vi "Create Subscription.vi"(7 "Inbound Message":refnum<user-event>, 8 "error in (no error)":errorcluster, 9 "SessionMailbox":refnum<queue>, 10 "QoS":T1, 11 "Topic Filter":string) -> (0 "error out":errorcluster, 3 "Subscription out":refnum<class "Subscription.lvclass">)   [LabVIEW 2013, in "MQTT Base.lvlib" / "Subscription.lvclass"]
uses:
  Subscription.lvclass
  <vilib>/LabVIEW Open Source Project/MQTT Control Packets/Control Packets/ControlPacket/QualityOfService -- enum.ctl
  Base Class/Response -- cluster.ctl
  <vilib>/LabVIEW Open Source Project/MQTT Control Packets/Control Packets/ControlPacket/ControlPacket.lvclass
  <vilib>/LabVIEW Open Source Project/MQTT Control Packets/Control Packets/PUBLISH/PUBLISH.lvclass
  Queued Message -- cluster.ctl
  Subscription.lvclass/Subscription.ctl
  TopicFilter/TopicFilter.lvclass
  Base Class/MQTT_Base.lvclass
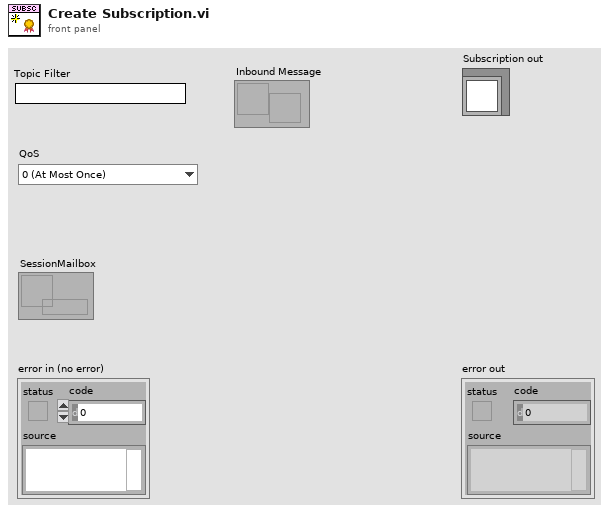
[diagram p1: front panel]
types:
  T1 = typedef "MQTT_Control_Packets.lvlib/ControlPacket.lvclass/QualityOfService -- enum.ctl" = enum16{"0 (At Most Once)", "1 (At Least Once)", "2 (Exactly Once)"}
  T2 = typedef "MQTT Base.lvlib/Subscription.lvclass/Queued Message -- cluster.ctl" = cluster{"Message":refnum<class "PUBLISH.lvclass">, "PUBREC received":bool}
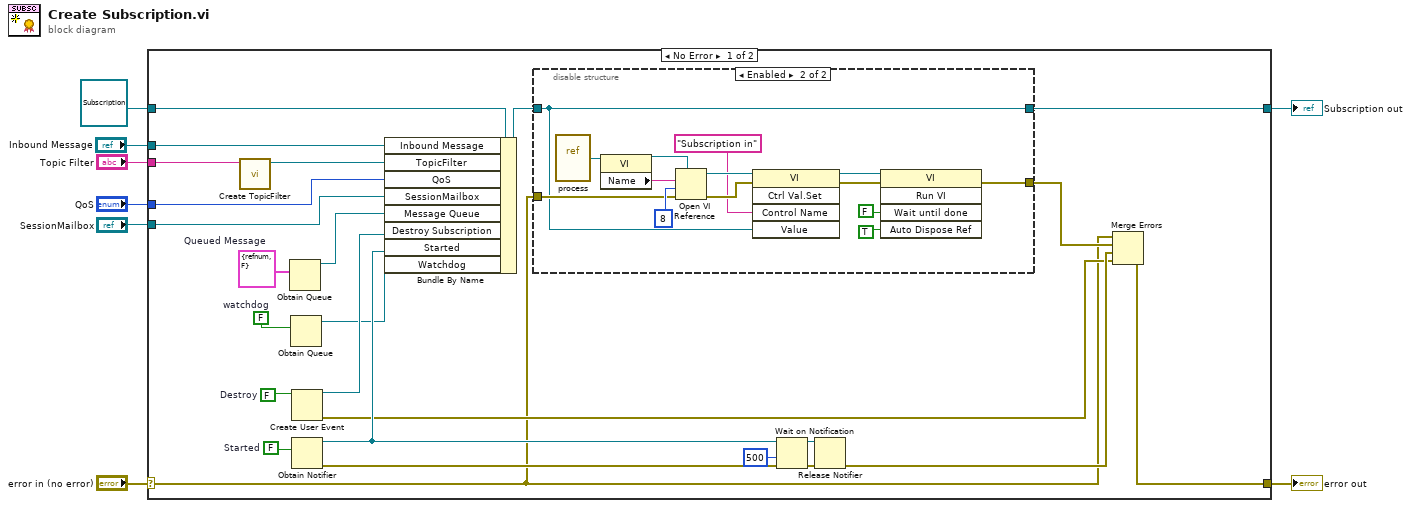
[diagram p0: block diagram]
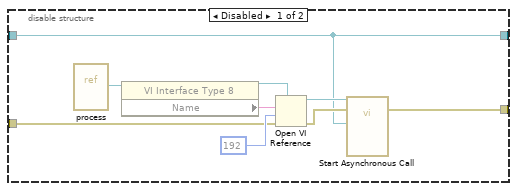
[diagram p2: hidden frame]
diagram:
  n1 = case shown="No Error" "error in (no error)" {
    selector: "error in (no error)" -> [w11 w58]
    tunnel: [w20 w58] -> w7
    tunnel: [w12 w57] -> w5
    tunnel: refnum<class "Subscription.lvclass"> refnum ("Subscription in") -> [w31 w57]
    tunnel: "Topic Filter" -> [w19 _]
    tunnel: "QoS" -> [w33 _]
    tunnel: "SessionMailbox" -> [w32 _]
    tunnel: "Inbound Message" -> [w29 _]
    frame No Error {
      w10 = FALSE  # watchdog
      w17 = FALSE  # Destroy
      w28 = FALSE  # Started
      w30 = T2 {"Message"=refnum, "PUBREC received"=FALSE}  # Queued Message
      n2 = call "Create TopicFilter.vi"("Topic Filter"=w19) -> ("TopicFilter out"=w18:refnum<class "TopicFilter.lvclass">)  [unwired: 9 in, 1 out]
      n3 = Obtain Queue(element data type=w30) -> (queue out=w27:refnum<queue>)  [unwired: 4 in, 2 out]
      n4 = Obtain Queue(element data type=w10) -> (queue out=w9:refnum<queue>)  [unwired: 4 in, 2 out]
      n5 = Create User Event(user event datatype=w17) -> (user event=w16:refnum<user-event>, error out=w15:errorcluster)  [unwired: 1 in]
      n6 = Obtain Notifier(notification data type=w28) -> (notifier out=w26:refnum<notifier>, error out=w23:errorcluster)  [unwired: 3 in, 1 out]
      n7 = Bundle By Name(cluster=w31, "Inbound Message"=w29, "TopicFilter"=w18, "QoS"=w33, "SessionMailbox"=w32, "Message Queue"=w27, "Destroy Subscription"=w16, "Started"=w26, "Watchdog"=w9) -> (w13:refnum<class "Subscription.lvclass">)
      n8 = disable-structure shown="Enabled" {
        disable-tunnel: w11 -> [w37 w53]
        disable-tunnel: w13 -> [w35 w46]
        disable-tunnel: [w36 w50] -> w14
        disable-tunnel: [w35 w46] -> w12
        frame Disabled {
          n9 = vi-ref "process.vi"() -> (w34:refnum<vi>)
          n10 = property class="VI Interface Type 8"(reference=w34) -> (reference out=w41:refnum<vi>, "Name"=w42:string)  [unwired: 1 in, 1 out]
          n11 = Open VI Reference(type specifier VI Refnum (for type only)=w41, vi path=w42, options=192, error in (no error)=w37) -> (vi reference=w40:refnum<vi>, error out=w39:errorcluster)  [unwired: 2 in]
          n12 = call-by-ref "Start Asynchronous Call"(reference=w40, error in=w39, "Subscription in"=w35) -> (error out=w36:errorcluster)  [unwired: 11 in, 1 out]
        }
        frame Enabled {
          n13 = vi-ref "process.vi"() -> (w43:refnum<vi>)
          n14 = property class="VI"(reference=w43) -> (reference out=w55:refnum<vi>, "Name"=w56:string)  [unwired: 1 in, 1 out]
          n15 = Open VI Reference(type specifier VI Refnum (for type only)=w55, vi path=w56, options=8, error in (no error)=w53) -> (vi reference=w48:refnum<vi>, error out=w49:errorcluster)  [unwired: 2 in]
          n16 = invoke class="VI" method="Ctrl Val.Set"(reference=w48, error in=w49, "Control Name"="Subscription in", "Value"=w46) -> (reference out=w45:refnum<vi>, error out=w44:errorcluster)  [unwired: 1 in, 3 out]
          n17 = invoke class="VI" method="Run VI"(reference=w45, error in=w44, "Wait until done"=FALSE ("Wait Until Done"), "Auto Dispose Ref"=TRUE ("Auto Dispose Reference")) -> (error out=w50:errorcluster)  [unwired: 1 in, 4 out]
        }
      }
      n18 = Wait on Notification(notifier=w26, timeout in ms (-1)=500, error in (no error)=w23) -> (notifier out=w24:refnum<notifier>, error out=w22:errorcluster)  [unwired: 1 in, 2 out]
      n19 = Release Notifier(notifier=w24, error in (no error)=w22) -> (error out=w21:errorcluster)  [unwired: 1 in, 2 out]
      n20 = Merge Errors(w11, w14, w21, w15) -> (w20:errorcluster)
    }
    frame Error {
    }
  }
  "error out" <- w7
  "Subscription out" <- w5
